vi "setWeatherData.vi"(8 "error in (no error)":errorcluster, 9 "WeatherData":T1, 11 "WeatherData in":refnum<class "Weather Station.lvclass">) -> (0 "error out":errorcluster, 3 "WeatherData out":refnum<class "Weather Station.lvclass">)   [LabVIEW 2020, in "Weather Station.lvclass"]
uses:
  Weather Station.lvclass
  Weather Station.lvclass/Weather Station.ctl
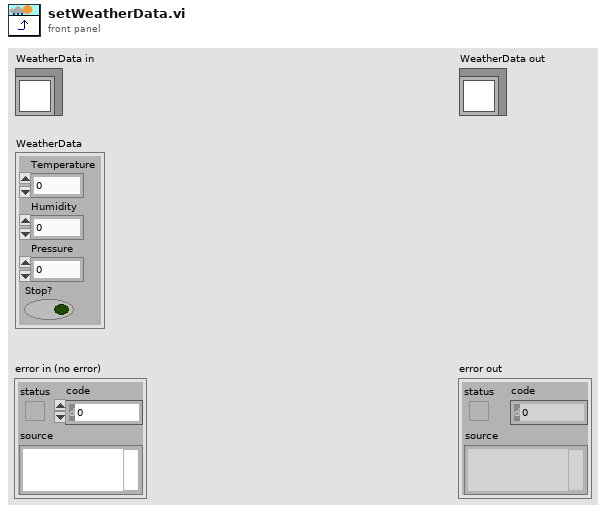
[diagram p1: front panel]
types:
  T1 = cluster{"Temperature":dbl, "Humidity":dbl, "Pressure":dbl, "Stop?":bool}
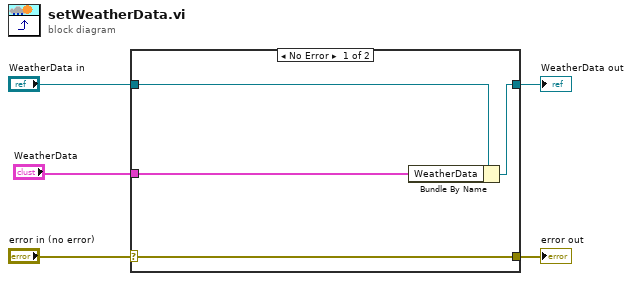
[diagram p0: block diagram]
diagram:
  n1 = case shown="No Error" "error in (no error)" {
    selector: "error in (no error)" -> [w9 w10]
    tunnel: [w9 w10] -> w4
    tunnel: [w7 w11] -> w2
    tunnel: "WeatherData in" -> [w8 w11]
    tunnel: "WeatherData" -> [w6 _]
    frame No Error {
      n2 = Bundle By Name(cluster=w8, "WeatherData"=w6) -> (w7:refnum<class "Weather Station.lvclass">)
    }
    frame Error {
    }
  }
  "error out" <- w4
  "WeatherData out" <- w2
